vi "Library Folder Children Data.vi"(7 "Destination":path=path "", 8 "Error In":errorcluster, 11 "Library In":refnum<vi>) -> (0 "Error Out":errorcluster, 2 "Data":refnum<class "Map.lvclass">[](array[class]), 3 "Library Out":refnum<vi>)   [LabVIEW 2018, in "Scripts.lvlib"]
uses:
  Scripts.lvlib
  Toolkit/Data/Map/Map.lvclass
  Toolkit/Data/Pair/Support/From String.vi
  Toolkit/Data/Map/Support/From Pair Array.vi
  Toolkit/Data/Pair/Pair.lvclass
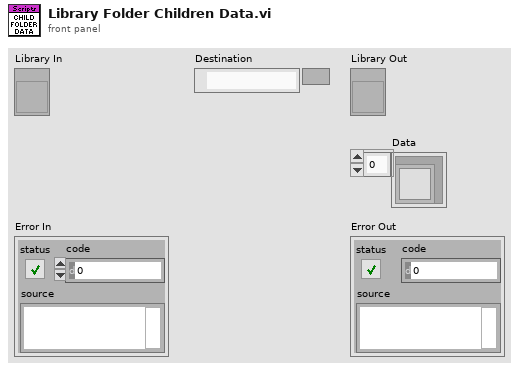
[diagram p1: front panel]
types:
  T1 = enum32{"invalid scope", "public", "private", "protected", "community"}
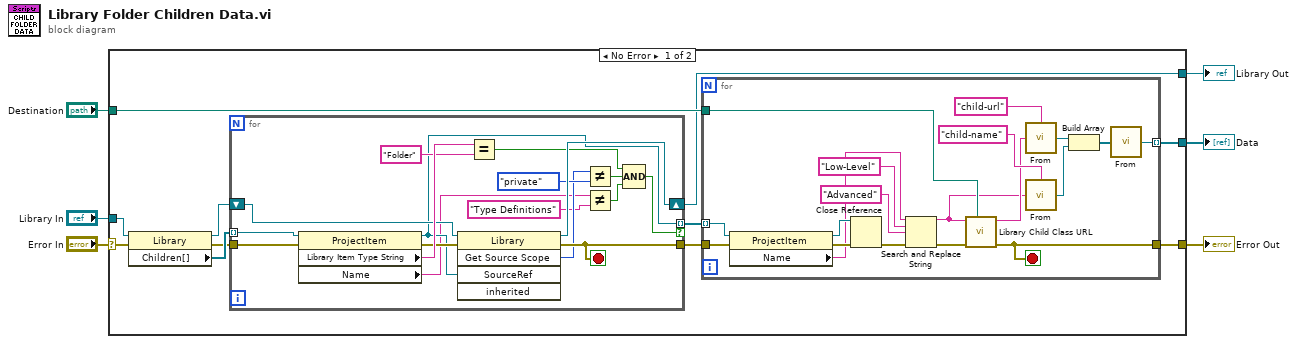
[diagram p0: block diagram]
diagram:
  n1 = case shown="No Error" "Error In" {
    selector: "Error In" -> [w13 w55]
    tunnel: [w17 w55] -> w6
    tunnel: "Destination" -> [w15 _]
    tunnel: "Library In" -> [w14 w54]
    tunnel: [w7 w54] -> w3
    tunnel: [w16 _] -> w2
    frame No Error {
      n2 = property class="Library"(reference=w14, error in=w13) -> (reference out=w8:refnum<vi>, error out=w11:errorcluster, "Children[]"=w12:refnum<vi>[])
      n3 = for {
        tunnel: w12 -> [w34] mode=indexing
        tunnel: w11 -> [w33]
        tunnel: [w26] -> w9 mode=indexing if=w19
        tunnel: [w27] -> w10
        shift-right: [w29] -> w7
        shift-left: w8 -> [w30]
        stop <- w27 stop-if-true
        n4 = property class="ProjectItem"(reference=w34, error in=w33) -> (reference out=w26:refnum<vi>, error out=w28:errorcluster, "Library Item Type String"=w32:string, "Name"=w23:string)
        n5 = invoke class="Library" method="Get Source Scope"(reference=w30, error in=w28, "SourceRef"=w26) -> (reference out=w29:refnum<vi>, error out=w27:errorcluster, "GetSourceScope"=w24:T1)  [unwired: 2 in, 2 out]
        n6 = Equal?(x=w32, y="Folder") -> (x = y?=w21:bool)
        n7 = Not Equal?(x=w24, y=T1."private" ("Source Scope:Get")) -> (x != y?=w20:bool)
        n8 = Not Equal?(x=w23, y="Type Definitions") -> (x != y?=w18:bool)
        n9 = Compound Arithmetic op=AND(w21, w20, w18) -> (w19:bool)
      }
      n10 = for {
        tunnel: w10 -> [w47]
        tunnel: [w48] -> w16 mode=indexing
        tunnel: [w42] -> w17
        tunnel: w15 -> [w43]
        tunnel: w9 -> [w41] mode=indexing
        stop <- w42 stop-if-true
        n11 = property class="ProjectItem"(reference=w41, error in=w47) -> (reference out=w45:refnum<vi>, error out=w46:errorcluster, "Name"=w40:string)
        n12 = Close Reference(reference=w45, error in (no error)=w46) -> (error out=w37:errorcluster)
        n13 = Search and Replace String(input string=w40, search string="Low-Level" ("substring (\"\")"), replace string="Advanced" ("replace string (\"\")"), error in=w37) -> (result string=w35:string, error out=w36:errorcluster)  [unwired: 4 in, 2 out]
        n14 = call "Library Child Class URL.vi"("Destination"=w43, "Error In"=w36, "Name"=w35) -> ("Error Out"=w42:errorcluster, "Child URL"=w44:string)  [unwired: 7 in]
        n15 = call-poly "From.vi"("Value"=w44, "Key"="child-url") -> ("Pair"=w51:refnum<class "Pair.lvclass">)
        n16 = call-poly "From.vi"("Value"=w35, "Key"="child-name") -> ("Pair"=w50:refnum<class "Pair.lvclass">)
        n17 = Build Array(w51, w50) -> (w49:refnum<class "Pair.lvclass">[])
        n18 = call-poly "From.vi"("Pairs"=w49) -> ("Map"=w48:refnum<class "Map.lvclass">)  [unwired: 1 in]
      }
    }
    frame Error {
    }
  }
  "Error Out" <- w6
  "Library Out" <- w3
  "Data" <- w2
